vi "HFRR ADV v014 new software.vi"() -> ()   [LabVIEW 2025] (continued)
            }
          }
        }
        n1459 = VISA Flush I/O Buffer(VISA resource name=w1688) -> (VISA resource name out=w1679:refnum<visa-resource-name>, error out=→"error out 9":errorcluster)  [unwired: 2 in]
        "Port 2a" <- TRUE ("Port 2a")
      }
      frame Error {
        w1729 = u16 0 items=["None", "XON/XOFF", "RTS/CTS", "XON/XOFF & RTS/CTS", "DTR/DSR", "XON/XOFF & DTR/DSR"] ("flow control (0:none)  2")
        w1727 = u16 10 items=["1.0"=10, "1.5"=15, "2.0"=20] ("stop bits 2")
        w1725 = u16 0 items=["None", "Odd", "Even", "Mark", "Space"] ("parity 2")
        w1726 = u32 10000  # timeout (10sec)
        n1460 = VISA Clear(VISA resource name=w1721, error in (no error)=w1718) -> (VISA resource name out=w1720:refnum<visa-resource-name>, error out=w1719:errorcluster)
        n1461 = VISA Close(VISA resource name=w1720, error in (no error)=w1719) -> (error out=w1722:errorcluster)
        n1462 = call <vilib>:"Clear Errors.vi"("error in (no error)"=w1722) -> ()  [unwired: 5 in, 2 out]
        n1463 = local write "Port 2a"(FALSE ("Port 2a")) -> ()
        n1464 = local read "Com Port 2"() -> (w1715:refnum<visa-resource-name>)
        "visa due" <- w1715
        n1465 = call-poly "VISA Configure Serial Port"("VISA resource name"=w1715, "timeout (10sec)"=w1726, "baud rate (9600)"=u32 250000 ("baud rate  2"), "data bits (8)"=u16 8 ("data bits  2"), "parity (0:none)"=w1725, "stop bits (10: 1 bit)"=w1727, "flow control (0:none)"=w1729) -> ("VISA resource name out"=w1730:refnum<visa-resource-name>, "error out"=w1731:errorcluster)  [unwired: 7 in]
        n1466 = flat-sequence {
          tunnel: w1730 -> [w1733]
          tunnel: w1731 -> [w1732]
          tunnel: [w1733] -> w1723
          tunnel: [w1732] -> w1716
          frame #0 {
            n1467 = Wait (ms)(milliseconds to wait=u32 50) -> ()  [unwired: 1 out]
          }
        }
        "Residual Due" <- ""
        "Port 2 Error" <- w1716
      }
    }
    n1468 = local read "Quit"() -> (w1658:bool)
    "Error Due" <- w1663
  }
  n1469 = local write "FRICVALZ"(0.0 ("FRICVALZ")) -> ()
  n1470 = property on="RUN" class="Bool (strict)"("Visible"=TRUE) -> ()  [unwired: 2 in, 2 out]
  n1471 = while {
    tunnel: [w1750] -> _
    tunnel: [w1735] -> w54
    i -> [w1750]
    stop <- w1735 stop-if-true
    n1472 = local read "conststatus"() -> (w1739:dbl)
    n1473 = local read "Main Tab"() -> (w1737:T2)
    n1474 = local read "EDIT"() -> (w1756:bool)
    n1475 = local read "Rate"() -> (w1755:dbl)
    n1476 = case shown="True" w1756 {
      tunnel: [FALSE TRUE] -> w1742
      frame False {
      }
      frame True {
      }
    }
    n1477 = property on="Time slide" class="Slide (strict)"("Scale.Range:Maximum"=2500.0) -> ()  [unwired: 2 in, 2 out]
    n1478 = Equal?(x=w1737, y=T27."About" ("Main Tab")) -> (x = y?=w1748:bool)
    n1479 = Equal?(x=w1739, y=0.0) -> (x = y?=w1740:bool)
    n1480 = Divide(x=1.0, y=w1755) -> (x/y=w1751:dbl)
    "Time 2" <- w1751
    n1481 = case shown="True" w1740 {
      frame False {
      }
      frame True {
        # "C:\\WinDucom\\calibrate WO 2391.dcf"
        n1482 = local write "Lan flag"(22) -> ()
        n1483 = local write "conststatus"(10.0 ("rpm value : 2")) -> ()
        n1484 = String To Path(string="C:\\LAB-IQ\\calibrate WO 2465.dcf") -> (path=w1762:path)
        n1485 = Open/Create/Replace File "Open File"(file path (use dialog)=w1762) -> (refnum out=w1760:refnum<file>)  [unwired: 5 in, 2 out]
        n1486 = for {
          N: 23 -> [_]
          tunnel: w1760 -> [w1771]
          i -> [w1765]
          (unwired) TRUE ("line mode (F)")
          n1487 = Read from Text File "Read File"(file (use dialog)=w1771) -> (text=w1770:string)  [unwired: 3 in, 3 out]
          n1488 = Match Pattern(string=w1770, regular expression="]") -> (after substring=w1768:string)  [unwired: 1 in, 3 out]
          n1489 = String Subset(string=w1770, offset (0)=5, length (rest)=10 ("length (rest)")) -> (substring=w1763:string)
          n1490 = Fract/Exp String To Number(string=w1763) -> (number=w1764:dbl)  [unwired: 3 in, 1 out]
          n1491 = Match Pattern(string=w1768, regular expression="-") -> (before substring=w1766:string)  [unwired: 1 in, 3 out]
          n1492 = case shown="19" w1765 {
            tunnel: w1764 -> [w1774 w1775 w1776 w1777 _ _ _ w1782 w1783 _ w1784 w1785 w1786 w1787 w1788 w1789 _ w1790 w1791 _ _ _ _ _]
            tunnel: w1766 -> [_ _ _ _ w1778 w1779 w1780 _ _ _ _ _ _ _ _ _ _ _ _ w1792 w1793 w1794 w1795 _]
            frame 0 {
              n1493 = local write "FRIC. FORCE :"(w1774) -> ()
            }
            frame 1 {
              n1494 = local write "TEMPERATURE :"(w1775) -> ()
            }
            frame 2 {
              n1495 = local write "HUMIDITY:"(w1776) -> ()
            }
            frame 3 {
              n1496 = local write "AIR TEMPERATURE :"(w1777) -> ()
            }
            frame 4 {
              n1497 = local write "Com Port 1"(w1778) -> ()
            }
            frame 5 {
              n1498 = local write "Com Port 2"(w1779) -> ()
              n1499 = local write "visa due"(w1779) -> ()
            }
            frame 6 {
              n1500 = String To Path(string=w1780) -> (path=w1781:path)
              n1501 = local write "File Path"(w1781) -> ()
              "String" <- w1780
            }
            frame 7 {
              n1502 = local write "DISPLACEMENT :"(w1782) -> ()
            }
            frame 8 {
              n1503 = local write "STROKE GAIN :"(w1783) -> ()
            }
            frame 9 {
            }
            frame 10 {
              n1504 = local write "Language Selection"(w1784) -> ()
            }
            frame 11 {
              n1505 = local write "CH-POWER +"(w1785) -> ()
            }
            frame 12 {
              n1506 = local write "CH-POWER -"(w1786) -> ()
            }
            frame 13 {
              n1507 = local write "CH-HEATER"(w1787) -> ()
            }
            frame 14 {
              n1508 = local write "CH-HUMIDITY WET"(w1788) -> ()
            }
            frame 15 {
              n1509 = local write "CH-HUMIDITY DRY"(w1789) -> ()
            }
            frame 16 {
            }
            frame 17 {
              n1510 = local write "AIR TEMP INTERCEPT:"(w1790) -> ()
            }
            frame 18 {
              n1511 = local write "TEMP INTERCEPT:"(w1791) -> ()
            }
            frame 21 {
              n1512 = local write "S.NO"(w1792) -> ()
            }
            frame 22 {
              n1513 = local write "Com Port 3"(w1793) -> ()
            }
            frame 20 {
              n1514 = local write "Camera Port :"(w1794) -> ()
            }
            frame 19 {
              n1515 = local write "C3 :"(w1795) -> ()
            }
            frame 23, Default {
            }
          }
        }
      }
    }
    n1516 = Select(t=u32 2500 ("milliseconds to wait"), s=w1748, f=u32 500 ("milliseconds to wait")) -> (s? t:f=w1746:u32)
    n1517 = Multiply(x=w1751, y=w1746) -> (x*y=w1753:dbl)
    n1518 = property on="Time slide" class="Slide (strict)"("Visible"=w1742) -> ()  [unwired: 2 in, 2 out]
    n1519 = call "Elapsed Time2"("Time Target (s)"=w1753, "Auto Reset"=TRUE) -> ("Time has Elapsed"=w1743:bool)  [unwired: 10 in, 7 out]
    n1520 = case shown="True" w1743 {
      frame False {
      }
      frame True {
        n1521 = stacked-sequence {
          frame #0 {
            # "DATA PROCESSING"
            # "115 mV/N"
            n1522 = local read "Sample Temperature"() -> (w1798:dbl)
            n1523 = local read "RH Numeric:"() -> (w1805:dbl)
            n1524 = local read "HUMIDITY:"() -> (w1806:dbl)
            n1525 = local read "FRICVALZ"() -> (w1817:dbl)
            n1526 = local read "Friction"() -> (w1801:dbl)
            n1527 = Multiply(x=w1805, y=w1806) -> (x*y=→"Humidity ( %RH )" →"Hum" →"Hum 2":dbl)
            n1528 = call <vilib>:"Mean PtByPt.vi"("x"=w1798, "sample length"=100) -> ("mean"=w1797:dbl)  [unwired: 2 in, 1 out]
            "TEMP 2" <- w1797
            "TEMP 3" <- w1797
            n1529 = Subtract(x=w1801, y=w1817) -> (x-y=w1812:dbl)
            "FF 2" <- w1812
            "FF 4" <- w1812
            n1530 = local read "Ambient Temperature"() -> (→"AIR TEMP":dbl)
            n1531 = local read "TEMP"() -> (w1816:dbl)
            n1532 = local write "FF 3"(w1812) -> ()
            n1533 = Compound Arithmetic op=OR("FRICVALZ 4", "FRICVALZ 3", "FRICVALZ 2") -> (w1808:bool)
            n1534 = case shown="True" w1808 {
              tunnel: w1801 -> [_ w1823]
              frame False {
              }
              frame True {
                w1822 = FALSE ("FRICVALZ")
                n1535 = local write "FRICVALZ 3"(w1822) -> ()
                n1536 = local write "FRICVALZ 2"(w1822) -> ()
                n1537 = local write "FRICVALZ 4"(w1822) -> ()
                "FRICVALZ" <- w1823
              }
            }
            n1538 = Not A Number/Path/Refnum?(number/path/refnum=w1816) -> (NaN/Path/Refnum?=w1815:bool)
            n1539 = Not A Number/Path/Refnum?(number/path/refnum=w1812) -> (NaN/Path/Refnum?=w1814:bool)
            n1540 = Divide(x=w1812, y=1.96) -> (x/y=w1809:dbl)
            n1541 = Compound Arithmetic op=OR(w1815, w1814) -> (w1813:bool)
            n1542 = Not A Number/Path/Refnum?(number/path/refnum=w1809) -> (NaN/Path/Refnum?=w1810:bool)
            n1543 = case shown="True" w1813 {
              frame False {
              }
              frame True {
                n1544 = local write "TEMP"(0.0 ("TEMP")) -> ()
                n1545 = local write "FF 2"(0.0 ("FF 2")) -> ()
                n1546 = local write "reinit"(TRUE ("reinit")) -> ()
              }
            }
            n1547 = local write "TEMP"(w1797) -> ()
            n1548 = Select(t=0.0, s=w1810, f=w1809) -> (s? t:f=w1800:dbl)
            "COF 2" <- w1800
            n1549 = local write "COF 3"(w1800) -> ()
          }
        }
      }
    }
    n1550 = Wait (ms)(milliseconds to wait=u32 50) -> ()  [unwired: 1 out]
    n1551 = local read "Quit"() -> (w1735:bool)
    "Rate" <- 2500.0 ("No of Samples")
  }
  n1552 = while {
    tunnel: w57 -> [_]
    tunnel: [w1850] -> _
    tunnel: [w1826] -> w56
    i -> [w1850]
    stop <- w1826 stop-if-true
    # "C:\\LAB-IQ-NXT\\Scar View.exe"
    n1553 = local read "OK Button 16"() -> (w1839:bool)
    n1554 = local read "Main Tab"() -> (w1832:T2)
    n1555 = local read "service 3"() -> (w1833:bool)
    n1556 = local read "OPEN 6"() -> (w1835:bool)
    n1557 = local read "EDIT 2"() -> (w1837:bool)
    n1558 = flat-sequence {
      frame #0 {
        n1559 = local read "SAVE 2"() -> (w2452:bool)
        n1560 = stacked-sequence {
          frame #0 {
            n1561 = local read "EDIT"() -> (w2506:bool)
            n1562 = case shown="True" w2506 {
              tunnel: [u8 2 ("Disabled") u8 0 ("Disabled")] -> _
              frame False {
                w2508 = FALSE
                n1563 = local write "Password"("") -> ()
                n1564 = property on="SrvM CP" class="Bool (strict)"("Visible"=w2508) -> ()  [unwired: 2 in, 2 out]
                n1565 = property on="message" class="Str"("Visible"=w2508) -> ()  [unwired: 2 in, 2 out]
                n1566 = local write "x = y?"(w2508) -> ()
                n1567 = property on="Password" class="Str"("Visible"=w2508) -> ()  [unwired: 2 in, 2 out]
                n1568 = property on="ENTER THE NEW PASSWORD" class="Str"("Visible"=w2508) -> ()  [unwired: 2 in, 2 out]
                n1569 = property on="ENTER CURRENT PASSWORD" class="Str"("Visible"=w2508) -> ()  [unwired: 2 in, 2 out]
                n1570 = local write "SrvM CP"(w2508) -> ()
              }
              frame True {
                w2511 = TRUE
                n1571 = property on="SrvM CP" class="Bool (strict)"("Visible"=w2511) -> ()  [unwired: 2 in, 2 out]
                n1572 = property on="Password" class="Str"("Visible"=w2511) -> ()  [unwired: 2 in, 2 out]
              }
            }
            "dipl pwd" <- "@143$\n" ("dipl pwd")
          }
          frame #1 {
            # "Gain password"
            n1573 = String To Byte Array(string="ENTER CURRENT PASSWORD") -> (unsigned byte array=w2516:u8[])
            n1574 = Search 1D Array(1D array=w2516, element=u8 10) -> (index of element=w2519:i32)  [unwired: 1 in]
            n1575 = Index Array(array=w2516, index=w2519) -> (element=w2515:u8)
            n1576 = Equal?(x=w2515, y=10) -> (x = y?=w2513:bool)
            n1577 = case shown="True" w2513 {
              frame False {
                n1578 = property on="ENTER THE NEW PASSWORD" class="Str"("Visible"=FALSE) -> ()  [unwired: 2 in, 2 out]
              }
              frame True {
                # "password"
                # "change password logic"
                n1579 = local read "ENTER CURRENT PASSWORD"() -> (w2532:string)
                n1580 = local read "dipl pwd"() -> (w2526:string)
                n1581 = String To Byte Array(string=w2532) -> (unsigned byte array=w2534:u8[])
                n1582 = String To Byte Array(string=w2526) -> (unsigned byte array=w2527:u8[])
                n1583 = Array Size(array=w2534) -> (size(s)=w2531:i32)
                n1584 = Array Size(array=w2527) -> (size(s)=w2529:i32)
                n1585 = for {
                  N: w2531 -> [_]
                  tunnel: w2534 -> [w2558]
                  tunnel: [w2556] -> w2535 mode=indexing
                  tunnel: w2531 -> [w2550]
                  i -> [w2551]
                  n1586 = Decrement(x=w2550) -> (x-1=w2548:i32)
                  n1587 = Equal?(x=w2551, y=w2548) -> (x = y?=w2549:bool)
                  n1588 = Index Array(array=w2558, index=w2551) -> (element=w2552:u8)
                  n1589 = Number To Decimal String(number=w2552) -> (decimal integer string=w2557:string)  [unwired: 1 in]
                  n1590 = Select(t="", s=w2549, f="\r") -> (s? t:f=w2554:string)
                  n1591 = Concatenate Strings(w2557, w2554) -> (w2556:string)
                }
                n1592 = for {
                  N: w2529 -> [_]
                  tunnel: w2527 -> [w2546]
                  tunnel: [w2544] -> w2528 mode=indexing
                  tunnel: w2529 -> [w2541]
                  i -> [w2542]
                  n1593 = Decrement(x=w2541) -> (x-1=w2540:i32)
                  n1594 = Equal?(x=w2542, y=w2540) -> (x = y?=w2539:bool)
                  n1595 = Index Array(array=w2546, index=w2542) -> (element=w2545:u8)
                  n1596 = Number To Decimal String(number=w2545) -> (decimal integer string=w2543:string)  [unwired: 1 in]
                  n1597 = Select(t="", s=w2539, f="\r") -> (s? t:f=w2536:string)
                  n1598 = Concatenate Strings(w2543, w2536) -> (w2544:string)
                }
                n1599 = local read "string"() -> (w2533:string)
                n1600 = Concatenate Strings(w2528) -> (w2522:string)
                n1601 = Concatenate Strings(w2533) -> (w2530:string)
                n1602 = Concatenate Strings(w2535) -> (w2523:string)
                n1603 = Equal?(x=w2523, y=w2530) -> (x = y?=w2525:bool)
                n1604 = Equal?(x=w2523, y=w2522) -> (x = y?=w2521:bool)
                n1605 = Or(x=w2525, y=w2521) -> (x .or. y?=w2524:bool)
                n1606 = case shown="True" w2524 {
                  frame False {
                  }
                  frame True {
                    n1607 = property on="ENTER THE NEW PASSWORD" class="Str"("Visible"=TRUE) -> ()  [unwired: 2 in, 2 out]
                  }
                }
              }
            }
          }
          frame #2 {
            n1608 = String To Byte Array(string="ENTER THE NEW PASSWORD") -> (unsigned byte array=w2561:u8[])
            n1609 = Search 1D Array(1D array=w2561, element=u8 10) -> (index of element=w2565:i32)  [unwired: 1 in]
            n1610 = Index Array(array=w2561, index=w2565) -> (element=w2563:u8)
            n1611 = Equal?(x=w2563, y=10) -> (x = y?=w2560:bool)
            n1612 = case shown="False" w2560 {
              frame False {
              }
              frame True {
                n1613 = local write "EDIT"(FALSE) -> ()
                n1614 = local write "SrvM CP"(FALSE) -> ()
                n1615 = local read "ENTER THE NEW PASSWORD"() -> (w2568:string)
                n1616 = String To Byte Array(string=w2568) -> (unsigned byte array=w2573:u8[])
                n1617 = Array Size(array=w2573) -> (size(s)=w2570:i32)
                n1618 = for {
                  N: w2570 -> [_]
                  tunnel: w2573 -> [w2586]
                  tunnel: [w2583] -> w2575 mode=indexing
                  tunnel: w2570 -> [w2578]
                  i -> [w2576]
                  n1619 = Decrement(x=w2578) -> (x-1=w2579:i32)
                  n1620 = Equal?(x=w2576, y=w2579) -> (x = y?=w2580:bool)
                  n1621 = Index Array(array=w2586, index=w2576) -> (element=w2585:u8)
                  n1622 = Number To Decimal String(number=w2585) -> (decimal integer string=w2584:string)  [unwired: 1 in]
                  n1623 = Select(t="", s=w2580, f="\r") -> (s? t:f=w2577:string)
                  n1624 = Concatenate Strings(w2584, w2577) -> (w2583:string)
                }
                n1625 = local read "file path"() -> (w2567:path)
                n1626 = Concatenate Strings(w2575) -> (w2569:string)
                n1627 = Delete(path (use dialog)=w2567) -> (deleted path=w2571:path)  [unwired: 4 in, 2 out]
                n1628 = call <vilib>:"Write Characters To File.vi"("append to file? (new file:F)"=FALSE, "character string"=w2569, "file path (dialog if empty)"=w2571) -> ()  [unwired: 2 in, 1 out]
              }
            }
          }
          frame #3 {
            n1629 = case shown="True" "SrvM CP" {
              frame False {
                w2589 = ""
                n1630 = local write "ENTER CURRENT PASSWORD"(w2589) -> ()
                n1631 = local write "ENTER THE NEW PASSWORD"(w2589) -> ()
                n1632 = property on="ENTER CURRENT PASSWORD" class="Str"("Visible"=FALSE) -> ()  [unwired: 2 in, 2 out]
              }
              frame True {
                n1633 = property on="ENTER THE NEW PASSWORD" class="Str"() -> ("Visible"=w2590:bool)  [unwired: 2 in, 2 out]
                n1634 = Not(x=w2590) -> (.not. x?=w2591:bool)
                n1635 = property on="ENTER CURRENT PASSWORD" class="Str"("Visible"=w2591) -> ()  [unwired: 2 in, 2 out]
              }
            }
          }
          frame #4 {
            n1636 = String To Byte Array(string="Password") -> (unsigned byte array=w2598:u8[])
            n1637 = Search 1D Array(1D array=w2598, element=u8 10) -> (index of element=w2596:i32)  [unwired: 1 in]
            n1638 = Index Array(array=w2598, index=w2596) -> (element=w2597:u8)
            n1639 = Equal?(x=w2597, y=10) -> (x = y?=w2593:bool)
            n1640 = case shown="True" w2593 {
              frame False {
              }
              frame True {
                # "password"
                # "password"
                n1641 = local read "Password"() -> (w2611:string)
                n1642 = String To Byte Array(string=w2611) -> (unsigned byte array=w2614:u8[])
                n1643 = String To Byte Array(string="@143$\n") -> (unsigned byte array=w2600:u8[])
                n1644 = Array Size(array=w2614) -> (size(s)=w2609:i32)
                n1645 = Array Size(array=w2600) -> (size(s)=w2605:i32)
                n1646 = for {
                  N: w2609 -> [_]
                  tunnel: w2614 -> [w2648]
                  tunnel: [w2646] -> w2615 mode=indexing
                  tunnel: w2609 -> [w2643]
                  i -> [w2644]
                  n1647 = Decrement(x=w2643) -> (x-1=w2642:i32)
                  n1648 = Index Array(array=w2648, index=w2644) -> (element=w2647:u8)
                  n1649 = Equal?(x=w2644, y=w2642) -> (x = y?=w2641:bool)
                  n1650 = Number To Decimal String(number=w2647) -> (decimal integer string=w2645:string)  [unwired: 1 in]
                  n1651 = Select(t="", s=w2641, f="\r") -> (s? t:f=w2638:string)
                  n1652 = Concatenate Strings(w2645, w2638) -> (w2646:string)
                }
                n1653 = for {
                  N: w2605 -> [_]
                  tunnel: w2600 -> [w2659]
                  tunnel: [w2657] -> w2603 mode=indexing
                  tunnel: w2605 -> [w2654]
                  i -> [w2655]
                  n1654 = Decrement(x=w2654) -> (x-1=w2653:i32)
                  n1655 = Index Array(array=w2659, index=w2655) -> (element=w2658:u8)
                  n1656 = Equal?(x=w2655, y=w2653) -> (x = y?=w2652:bool)
                  n1657 = Number To Decimal String(number=w2658) -> (decimal integer string=w2656:string)  [unwired: 1 in]
                  n1658 = Select(t="", s=w2652, f="\r") -> (s? t:f=w2649:string)
                  n1659 = Concatenate Strings(w2656, w2649) -> (w2657:string)
                }
                n1660 = local read "file path"() -> (w2599:path)
                n1661 = call <vilib>:"Read Characters From File.vi"("file path (dialog if empty)"=w2599) -> ("character string"=w2613:string)  [unwired: 5 in, 3 out]
                "string" <- w2613
                n1662 = flat-sequence {
                  tunnel: [w2616] -> w2610
                  frame #0 {
                    w2616 = ""
                    n1663 = local write "Password"(w2616) -> ()
                  }
                }
                n1664 = Concatenate Strings(w2603) -> (w2604:string)
                n1665 = Concatenate Strings(w2613) -> (w2612:string)
                n1666 = Concatenate Strings(w2615) -> (w2607:string)
                n1667 = Equal?(x=w2607, y=w2612) -> (x = y?=w2602:bool)
                n1668 = Equal?(x=w2607, y=w2604) -> (x = y?=w2608:bool)
                n1669 = Or(x=w2602, y=w2608) -> (x .or. y?=w2601:bool)
                "x = y?" <- w2601
                n1670 = case shown="True" w2601 {
                  selector: w2601 -> [w2618 _]
                  tunnel: w2610 -> [_ _]
                  frame False {
                    n1671 = And(x=w2618, y=TRUE ("Visible")) -> (x .and. y?=w2619:bool)
                    n1672 = property on="message" class="Str"("Visible"=w2619) -> ()  [unwired: 2 in, 2 out]
                  }
                  frame True {
                    n1673 = control-ref of="This VI"() -> (w2630:refnum<vi>)
                    n1674 = property class="VI"(reference=w2630) -> (reference out=w2621:refnum<vi>, error out=w2625:errorcluster, "Panel"=w2629:refnum<vi>)  [unwired: 1 in]
                    n1675 = property on="message" class="Str"("Visible"=FALSE) -> ()  [unwired: 2 in, 2 out]
                    n1676 = property class="Pnl"(reference=w2629, error in=w2625) -> (reference out=w2623:refnum<vi>, error out=w2626:errorcluster, "Panes[]"=w2628:refnum<vi>[])
                    n1677 = for {
                      tunnel: w2628 -> [w2637] mode=indexing
                      tunnel: T21."Always On" ("Horizontal Scrollbar Visibility") -> [w2636]
                      tunnel: w2626 -> [w2633]
                      tunnel: [w2632] -> w2624
                      n1678 = property class="Pane"(reference=w2637, error in=w2633, "HorizScrollbarVisibility"=w2636) -> (reference out=w2634:refnum<vi>, error out=w2635:errorcluster)
                      n1679 = Close Reference(reference=w2634, error in (no error)=w2635) -> (error out=w2632:errorcluster)
                    }
                    n1680 = Close Reference(reference=w2623, error in (no error)=w2624) -> (error out=w2622:errorcluster)
                    n1681 = Close Reference(reference=w2621, error in (no error)=w2622) -> (error out=→"error out 6":errorcluster)
                  }
                }
              }
            }
          }
        }
        n1682 = local read "x = y?"() -> (w2458:bool)
        n1683 = local read "HUMIDITY: 2"() -> (w2460:dbl)
        n1684 = local read "HUMIDITY:"() -> (w2459:dbl)
        n1685 = property on="Port 2 Error" class="Clust (strict)"("Visible"="EDIT") -> ()  [unwired: 2 in, 2 out]
        n1686 = property on="Port 1 Error" class="Clust (strict)"("Visible"="EDIT") -> ()  [unwired: 2 in, 2 out]
        n1687 = case shown="True" "SrvM CP 2" {
          frame False {
          }
          frame True {
            n1688 = local write "SrvM CP 2"(FALSE ("SrvM CP 2")) -> ()
            n1689 = local read "HUMIDITY: 2"() -> (w2499:dbl)
            n1690 = local read "TEMP INTERCEPT: 2"() -> (w2498:dbl)
            n1691 = local read "DISPLACEMENT : 4"() -> (w2502:dbl)
            n1692 = local read "TEMPERATURE : 2"() -> (w2501:dbl)
            n1693 = local read "STROKE GAIN : 2"() -> (w2503:dbl)
            n1694 = local read "FRIC. FORCE : 2"() -> (w2504:dbl)
            n1695 = local read "AIR TEMP INTERCEPT: 2"() -> (w2497:dbl)
            n1696 = local read "AIR TEMPERATURE : 2"() -> (w2500:dbl)
            n1697 = local write "HUMIDITY:"(w2499) -> ()
            n1698 = local write "AIR TEMP INTERCEPT:"(w2498) -> ()
            n1699 = local write "TEMPERATURE :"(w2501) -> ()
            n1700 = local write "FRIC. FORCE :"(w2504) -> ()
            n1701 = local write "STROKE GAIN :"(w2503) -> ()
            n1702 = local write "DISPLACEMENT :"(w2502) -> ()
            n1703 = local write "AIR TEMPERATURE :"(w2500) -> ()
            n1704 = local write "TEMP INTERCEPT:"(w2497) -> ()
          }
        }
        n1705 = Or(x="SAVE", y=w2452) -> (x .or. y?=w2453:bool)
        n1706 = And(x="EDIT", y=w2458) -> (x .and. y?=w2456:bool)
        n1707 = local read "DISPLACEMENT : 4"() -> (w2469:dbl)
        n1708 = local read "TEMPERATURE : 2"() -> (w2467:dbl)
        n1709 = local read "STROKE GAIN : 2"() -> (w2473:dbl)
        n1710 = local read "DISPLACEMENT :"() -> (w2468:dbl)
        n1711 = local read "FRIC. FORCE : 2"() -> (w2476:dbl)
        n1712 = local read "TEMPERATURE :"() -> (w2465:dbl)
        n1713 = local read "STROKE GAIN :"() -> (w2472:dbl)
        n1714 = local read "FRIC. FORCE :"() -> (w2475:dbl)
        n1715 = case shown="True" w2456 {
          tunnel: [u8 2 ("Disabled") u8 0 ("Disabled")] -> w2455
          tunnel: [w2820 TRUE ("Visible")] -> w2454
          frame False {
            w2820 = FALSE ("Visible")
            n1716 = local write "EDIT 2"(w2820) -> ()
          }
          frame True {
          }
        }
        n1717 = case shown="True" w2453 {
          frame False {
          }
          frame True {
            n1718 = stacked-sequence {
              seq-local: [w2668 _ _] -> [_ w2815 _]
              frame #0 {
                (unwired) i16 5 ("precision (6)")
                # "[CH1]    - FF\n[CH2]   - TEMPERATURE\n[CH3]    - Humidity\n[CH4]    - AIR TEMP\n[CH5]\\- Visa Uno\n[CH6] \\- Visa Due\n[CH7]  \\- file path\n[CH8]   - Displacement Gain\n[CHA]   - Stroke Gain\n[CHB]   - Stroke PID Gain\n[CHC]   -Language Selection\n[CHD]   -Power +\n[CHE]   -Power_\n[CHF]   -Heater\n[CHG]   -Humidity Wet\n[CHH]   -Humidity Dry\n[CHI]   -Integral Time"
                n1719 = local read "Language Selection"() -> (w2716:enum16{"English", "Russian"})
                n1720 = local read "CH-HUMIDITY WET"() -> (w2674:u16)
                n1721 = local read "CH-HUMIDITY DRY"() -> (w2671:u16)
                n1722 = local read "STROKE GAIN :"() -> (w2660:dbl)
                n1723 = local read "CH-POWER +"() -> (w2683:u16)
                n1724 = local read "CH-POWER -"() -> (w2680:u16)
                n1725 = local read "CH-HEATER"() -> (w2677:u16)
                n1726 = local read "AIR TEMPERATURE :"() -> (w2663:dbl)
                n1727 = local read "DISPLACEMENT :"() -> (w2661:dbl)
                n1728 = local read "TEMPERATURE :"() -> (w2664:dbl)
                n1729 = local read "FRIC. FORCE :"() -> (w2665:dbl)
                n1730 = local read "HUMIDITY:"() -> (w2662:dbl)
                n1731 = Path To String(path="File Path") -> (string=w2732:string)
                n1732 = Number To Fractional String(number=w2660, width (-)=i16 10 ("precision (6)"), precision (6)=i16 5) -> (F-format string=w2723:string)  [unwired: 1 in]
                n1733 = Number To Fractional String(number=w2716, width (-)=i16 10 ("precision (6)"), precision (6)=i16 5) -> (F-format string=w2712:string)  [unwired: 1 in]
                n1734 = Number To Fractional String(number=w2683, width (-)=i16 10 ("precision (6)"), precision (6)=i16 5) -> (F-format string=w2706:string)  [unwired: 1 in]
                n1735 = Number To Fractional String(number=w2680, width (-)=i16 10 ("precision (6)"), precision (6)=i16 5) -> (F-format string=w2703:string)  [unwired: 1 in]
                n1736 = Number To Fractional String(number=w2677, width (-)=i16 10 ("precision (6)"), precision (6)=i16 5) -> (F-format string=w2698:string)  [unwired: 1 in]
                n1737 = Number To Fractional String(number=w2674, width (-)=i16 10 ("precision (6)"), precision (6)=i16 5) -> (F-format string=w2695:string)  [unwired: 1 in]
                n1738 = Number To Fractional String(number=w2671, width (-)=i16 10 ("precision (6)"), precision (6)=i16 5) -> (F-format string=w2690:string)  [unwired: 1 in]
                n1739 = local read "Com Port 1"() -> (w2667:refnum<visa-resource-name>)
                n1740 = local read "Com Port 2"() -> (w2666:refnum<visa-resource-name>)
                n1741 = Concatenate Strings(w2732, "\\" ("string")) -> (w2731:string)
                n1742 = Number To Fractional String(number=w2665, width (-)=i16 10 ("precision (6)"), precision (6)=i16 5) -> (F-format string=w2764:string)  [unwired: 1 in]
                n1743 = Number To Fractional String(number=w2664, width (-)=i16 10 ("precision (6)"), precision (6)=i16 5) -> (F-format string=w2763:string)  [unwired: 1 in]
                n1744 = Number To Fractional String(number=w2662, width (-)=i16 10 ("precision (6)"), precision (6)=i16 5) -> (F-format string=w2757:string)  [unwired: 1 in]
                n1745 = Number To Fractional String(number=w2663, width (-)=i16 10 ("precision (6)"), precision (6)=i16 5) -> (F-format string=w2751:string)  [unwired: 1 in]
                n1746 = Number To Fractional String(number=w2661, width (-)=i16 10 ("precision (6)"), precision (6)=i16 5) -> (F-format string=w2724:string)  [unwired: 1 in]
                n1747 = Concatenate Strings("[CHA]" ("string"), w2723, "- Stroke Gain" ("string"), "\r") -> (w2717:string)
                n1748 = Concatenate Strings("[CHC]" ("string"), w2712, "-Language Selection" ("string"), "\r") -> (w2709:string)
                n1749 = Concatenate Strings("[CHD]" ("string"), w2706, "-Power +" ("string"), "\r") -> (w2688:string)
                n1750 = Concatenate Strings("[CHG]" ("string"), w2695, "-Humidity Wet" ("string"), "\r") -> (w2685:string)
                n1751 = Concatenate Strings("[CHH]" ("string"), w2690, "-Humidity Dry" ("string"), "\r") -> (w2684:string)
                n1752 = Concatenate Strings("[CH1]" ("string"), w2764, " - FF" ("string"), "\r") -> (w2762:string)
                n1753 = Concatenate Strings("[CH2]" ("string"), w2763, " - TEMPERATURE" ("string"), "\r") -> (w2761:string)
                n1754 = Concatenate Strings("[CH3]" ("string"), w2757, " - Humidity" ("string"), "\r") -> (w2754:string)
                n1755 = Concatenate Strings("[CH4]" ("string"), w2751, " - AIR TEMP" ("string"), "\r") -> (w2747:string)
                n1756 = Concatenate Strings("[CH5]" ("string"), w2667, "- Visa Uno" ("string"), "\r") -> (w2740:string)
                n1757 = Concatenate Strings("[CH6]" ("string"), w2666, "- Visa Due" ("string"), "\r") -> (w2735:string)
                n1758 = Concatenate Strings("[CH7]" ("string"), w2731, "- file path" ("string"), "\r") -> (w2734:string)
                n1759 = Concatenate Strings("[CH8]" ("string"), w2724, "- Displacement Gain" ("string"), "\r") -> (w2727:string)
                n1760 = Concatenate Strings("[CHE]" ("string"), w2703, "-Power_" ("string"), "\r") -> (w2687:string)
                n1761 = Concatenate Strings("[CHF]" ("string"), w2698, "-Heater" ("string"), "\r") -> (w2686:string)
                n1762 = Concatenate Strings(w2762, w2761, w2754, w2747, w2740, w2735, w2734, w2727, w2717, w2709, w2688, w2687, w2686, w2685, w2684) -> (w2668:string)
                "gain" <- w2668
              }
              frame #1 {
                n1763 = local read "Camera Port :"() -> (w2776:string)
                n1764 = local read "C3 :"() -> (w2784:refnum<visa-resource-name>)
                n1765 = local read "TEMP INTERCEPT:"() -> (w2785:dbl)
                n1766 = local read "AIR TEMP INTERCEPT:"() -> (w2786:dbl)
                n1767 = local read "Com Port 3"() -> (w2787:refnum<visa-resource-name>)
                n1768 = Concatenate Strings("[CH8]" ("string"), w2776, "- Visa Camera" ("string"), "\r") -> (w2775:string)
                n1769 = Concatenate Strings("[CH7]" ("string"), w2784, "- Visa Humidity" ("string"), "\r") -> (w2780:string)
                n1770 = Number To Fractional String(number=w2785, width (-)=i16 10 ("precision (6)"), precision (6)=i16 5) -> (F-format string=w2803:string)  [unwired: 1 in]
                n1771 = Concatenate Strings("[CHL]" ("string"), w2787, "- Visa humid" ("string"), "\r") -> (w2790:string)
                n1772 = Number To Fractional String(number=w2786, width (-)=i16 10 ("precision (6)"), precision (6)=i16 5) -> (F-format string=w2810:string)  [unwired: 1 in]
                n1773 = Concatenate Strings("[CHK]" ("string"), w2803, "-TEMP INTERCEPT" ("string"), "\r") -> (w2799:string)
                n1774 = Concatenate Strings("[SNO]" ("string"), "S.NO", "-" ("string"), "\r") -> (w2795:string)
                n1775 = Concatenate Strings("[CHJ]" ("string"), w2810, "-AIR TEMP INTERCEPT" ("string"), "\r") -> (w2800:string)
                n1776 = String To Path(string="C:\\LAB-IQ\\calibrate WO 2465.dcf") -> (path=w2788:path)
                n1777 = Concatenate Strings(w2815, w2800, w2799, w2795, w2790, w2780, w2775) -> (w2814:string)
                n1778 = call <vilib>:"Write Characters To File.vi"("append to file? (new file:F)"=FALSE, "character string"=w2814, "file path (dialog if empty)"=w2788) -> ()  [unwired: 2 in, 1 out]
              }
              frame #2 {
                n1779 = local write "Lan flag"(0.0 ("Lan flag")) -> ()
                n1780 = local write "conststatus"(0.0 ("rpm value : 2")) -> ()
                n1781 = local write "SAVE"(FALSE ("OK Button 14")) -> ()
                n1782 = local write "SAVE 2"(FALSE ("SAVE 2")) -> ()
              }
            }
          }
        }
        n1783 = Subtract(x=w2460, y=w2459) -> (x-y=w2461:dbl)
        n1784 = local read "AIR TEMPERATURE : 2"() -> (w2464:dbl)
        n1785 = local read "AIR TEMPERATURE :"() -> (w2463:dbl)
        n1786 = Divide(x=w2461, y=w2459) -> (x/y=w2483:dbl)
        n1787 = Subtract(x=w2476, y=w2475) -> (x-y=w2474:dbl)
        n1788 = Subtract(x=w2467, y=w2465) -> (x-y=w2466:dbl)
        n1789 = Subtract(x=w2473, y=w2472) -> (x-y=w2471:dbl)
        n1790 = Subtract(x=w2469, y=w2468) -> (x-y=w2470:dbl)
        n1791 = Subtract(x=w2464, y=w2463) -> (x-y=w2462:dbl)
        n1792 = Divide(x=w2474, y=w2475) -> (x/y=w2494:dbl)
        n1793 = Divide(x=w2466, y=w2465) -> (x/y=w2487:dbl)
        n1794 = Divide(x=w2471, y=w2472) -> (x/y=w2491:dbl)
        n1795 = Divide(x=w2470, y=w2468) -> (x/y=w2490:dbl)
        n1796 = Multiply(x=w2483, y=100.0) -> (x*y=→"HUMIDITY  Calibration Error":dbl)
        n1797 = Divide(x=w2462, y=w2463) -> (x/y=w2486:dbl)
        n1798 = Multiply(x=w2494, y=100.0) -> (x*y=→"FRIC. FORCE Calibration Error":dbl)
        n1799 = Multiply(x=w2487, y=100.0) -> (x*y=→"TEMPERATURE  Calibration Error":dbl)
        n1800 = Multiply(x=w2491, y=100.0) -> (x*y=→"STROKE Calibration Error":dbl)
        n1801 = Multiply(x=w2490, y=100.0) -> (x*y=→"DISPLACEMENT  Calibration Error":dbl)
        n1802 = property on="EDIT 2" class="Bool (strict)"("Visible"=w2454) -> ()  [unwired: 2 in, 2 out]
        n1803 = property on="SAVE" class="Bool (strict)"("Visible"=w2454) -> ()  [unwired: 2 in, 2 out]
        n1804 = property on="SrvM CP" class="Bool (strict)"("Disabled"=w2455) -> ()  [unwired: 2 in, 2 out]
        n1805 = property on="visa due" class="CmbBox"("Disabled"=w2455) -> ()  [unwired: 2 in, 2 out]
        n1806 = property on="File Path" class="Path"("Disabled"=w2455) -> ()  [unwired: 2 in, 2 out]
        n1807 = Multiply(x=w2486, y=100.0) -> (x*y=→"AIR TEMPERATURE  Calibration Error":dbl)
        n1808 = property on="Language Selection" class="Enum (strict)"("Visible"=w2454) -> ()  [unwired: 2 in, 2 out]
        n1809 = property on="Tab Control 7" class="TabCtl (strict)"("Disabled"=w2455) -> ()  [unwired: 2 in, 2 out]
        n1810 = property on="AIR TEMP INTERCEPT:" class="DigNum (strict)"("Disabled"=w2455) -> ()  [unwired: 2 in, 2 out]
        n1811 = property on="CH-POWER -" class="DigNum (strict)"("Disabled"=w2455) -> ()  [unwired: 2 in, 2 out]
        n1812 = property on="CH-POWER +" class="DigNum (strict)"("Disabled"=w2455) -> ()  [unwired: 2 in, 2 out]
        n1813 = property on="AIR TEMPERATURE :" class="DigNum (strict)"("Disabled"=w2455) -> ()  [unwired: 2 in, 2 out]
        n1814 = property on="STROKE GAIN :" class="DigNum (strict)"("Disabled"=w2455) -> ()  [unwired: 2 in, 2 out]
        n1815 = property on="SPEED OUT:" class="DigNum (strict)"("Disabled"=w2455) -> ()  [unwired: 2 in, 2 out]
        n1816 = property on="CH-HUMIDITY DRY" class="DigNum (strict)"("Disabled"=w2455) -> ()  [unwired: 2 in, 2 out]
        n1817 = property on="HUMIDITY:" class="DigNum (strict)"("Disabled"=w2455) -> ()  [unwired: 2 in, 2 out]
        n1818 = property on="CH-HUMIDITY WET" class="DigNum (strict)"("Disabled"=w2455) -> ()  [unwired: 2 in, 2 out]
        n1819 = property on="TEMPERATURE :" class="DigNum (strict)"("Disabled"=w2455) -> ()  [unwired: 2 in, 2 out]
        n1820 = property on="DISPLACEMENT :" class="DigNum (strict)"("Disabled"=w2455) -> ()  [unwired: 2 in, 2 out]
        n1821 = property on="CH-HEATER" class="DigNum (strict)"("Disabled"=w2455) -> ()  [unwired: 2 in, 2 out]
        n1822 = property on="TEMP INTERCEPT:" class="DigNum (strict)"("Disabled"=w2455) -> ()  [unwired: 2 in, 2 out]
        n1823 = property on="FRIC. FORCE :" class="DigNum (strict)"("Disabled"=w2455) -> ()  [unwired: 2 in, 2 out]
      }
    }
    n1824 = local read "RUN"() -> (w1849:bool)
    n1825 = local read "RUN"() -> (w1847:bool)
    n1826 = disable-structure shown="Disabled" {
      disable-tunnel: [w1864 _] -> w1830
      disable-tunnel: [w1863 _] -> w1828
      frame Disabled {
        n1827 = local read "Temperature before test"() -> (w1857:dbl)
        n1828 = local read "Temperature after test"() -> (w1870:dbl)
        n1829 = case shown="True" "Save Results" {
          frame False {
          }
          frame True {
            w1886 = "\r"
            n1830 = local write "Save Results"(FALSE ("OK Button 5")) -> ()
            n1831 = local read "Temperature before test"() -> (w1924:dbl)
            n1832 = local read "Temperature after test"() -> (w1926:dbl)
            n1833 = local read "Humidity before test"() -> (w1923:dbl)
            n1834 = local read "Humidity after test"() -> (w1925:dbl)
            n1835 = local read "WS1.4"() -> (w1930:dbl)
            n1836 = local read "AVP"() -> (w1928:dbl)
            n1837 = Number To Fractional String(number=w1930, width (-)=i16 6, precision (6)=i16 1) -> (F-format string=w1890:string)  [unwired: 1 in]
            n1838 = local read "MWSD"() -> (w1927:dbl)
            n1839 = local read "String"() -> (w1919:string)
            n1840 = local read "FILE"() -> (w1922:string)
            n1841 = local read "HCF"() -> (w1929:dbl)
            n1842 = Number To Fractional String(number=w1923, width (-)=i16 6, precision (6)=i16 1) -> (F-format string=w1915:string)  [unwired: 1 in]
            n1843 = Number To Fractional String(number=w1924, width (-)=i16 6, precision (6)=i16 1) -> (F-format string=w1912:string)  [unwired: 1 in]
            n1844 = Number To Fractional String(number=w1925, width (-)=i16 6, precision (6)=i16 1) -> (F-format string=w1908:string)  [unwired: 1 in]
            n1845 = Number To Fractional String(number=w1926, width (-)=i16 6, precision (6)=i16 1) -> (F-format string=w1904:string)  [unwired: 1 in]
            n1846 = Number To Fractional String(number=w1928, width (-)=i16 6, precision (6)=i16 3) -> (F-format string=w1897:string)  [unwired: 1 in]
            n1847 = Concatenate Strings(w1919, w1922) -> (w1941:string)
            n1848 = Number To Fractional String(number=w1927, width (-)=i16 6, precision (6)=i16 1) -> (F-format string=w1901:string)  [unwired: 1 in]
            n1849 = Number To Fractional String(number=w1929, width (-)=i16 6, precision (6)=i16 2) -> (F-format string=w1895:string)  [unwired: 1 in]
            n1850 = Concatenate Strings("(" ("string"), w1890, ")Microns" ("string")) -> (w1889:string)
            n1851 = local read "REMARKS"() -> (w1921:string)
            "REMARKS 2" <- w1921
            n1852 = Concatenate Strings("(" ("string"), w1915, " ) % RH," ("string")) -> (w1916:string)
            n1853 = Concatenate Strings(w1895, ")" ("string")) -> (w1893:string)
            n1854 = Concatenate Strings("(" ("string"), w1912, ")  Deg C ," ("string")) -> (w1911:string)
            n1855 = Concatenate Strings("(" ("string"), w1908, " ) % RH," ("string")) -> (w1907:string)
            n1856 = Concatenate Strings("(" ("string"), w1904, ")  Deg C ," ("string")) -> (w1903:string)
            n1857 = Concatenate Strings("(" ("string"), w1901, ")  Microns," ("string")) -> (w1900:string)
            n1858 = Concatenate Strings("(" ("string"), w1897, ")  kPa," ("string")) -> (w1887:string)
            n1859 = Concatenate Strings(w1941, ".dwm" ("Substring")) -> (w1939:string)
            n1860 = String To Path(string=w1939) -> (path=w1938:path)
            n1861 = Concatenate Strings(w1921, w1886, " Humidity before test= " ("Substring"), w1916, w1886, " Temperature before test = " ("Substring"), w1911, w1886, " Humidity after test= " ("Substring"), w1907, w1886, "Temperature after test = " ("Substring"), w1903, w1886, "MSD = " ("Substring"), w1900, w1886, "  AVP = " ("Substring"), w1887, w1886, "  HCF                     =( " ("Substring"), w1893, w1886, " WS1.4                  = " ("Substring"), w1889, w1886) -> (w1885:string)
            "data" <- w1885
            n1862 = call <vilib>:"Write Characters To File.vi"("append to file? (new file:F)"=FALSE, "character string"=w1885, "file path (dialog if empty)"=w1938) -> ()  [unwired: 2 in, 1 out]
            n1863 = Match Pattern(string=w1885, regular expression="!") -> (after substring=→"export":string)  [unwired: 1 in, 3 out]
          }
        }
        n1864 = Add(x=231.864, y=w1857) -> (x+y=w1854:dbl)
        n1865 = Add(x=231.864, y=w1870) -> (x+y=w1867:dbl)
        n1866 = Divide(x=1705.984, y=w1854) -> (x/y=w1855:dbl)
        n1867 = Divide(x=1705.984, y=w1867) -> (x/y=w1868:dbl)
        n1868 = local read "Humidity before test"() -> (w1859:dbl)
        n1869 = local read "Humidity after test"() -> (w1872:dbl)
        n1870 = Subtract(x=8.017352 ("y"), y=w1855) -> (x-y=w1881:dbl)
        n1871 = Subtract(x=8.017352 ("y"), y=w1868) -> (x-y=w1875:dbl)
        n1872 = expression code="10**y"(w1881) -> (w1861:dbl)
        n1873 = expression code="10**y"(w1875) -> (w1874:dbl)
        n1874 = Multiply(x=w1859, y=w1861) -> (x*y=w1860:dbl)
        n1875 = Multiply(x=w1872, y=w1874) -> (x*y=w1873:dbl)
        n1876 = Divide(x=w1860, y=750.0) -> (x/y=w1876:dbl)
        n1877 = Divide(x=w1873, y=750.0) -> (x/y=w1877:dbl)
        n1878 = Add(x=w1876, y=w1877) -> (x+y=w1878:dbl)
        n1879 = Divide(x=w1878, y=2.0) -> (x/y=w1880:dbl)
        n1880 = local write "AVP"(w1880) -> ()
        n1881 = Subtract(x=1.4, y=w1880) -> (x-y=w1863:dbl)
        n1882 = local read "HCF"() -> (w1864:dbl)
      }
      frame Enabled {
      }
    }
    n1883 = case shown="True" "EDIT 3" {
      frame False {
      }
      frame True {
        n1884 = local write "EDIT 3"(FALSE ("EDIT 3")) -> ()
        n1885 = local write "Main Tab"(T2."About" ("Main Tab")) -> ()
      }
    }
    n1886 = case shown="False" w1849 {
      frame False {
        n1887 = local read "stopT"() -> (w2827:bool)
        n1888 = case shown="True" w2827 {
          frame False {
          }
          frame True {
            n1889 = local write "stopT"(FALSE) -> ()
          }
        }
      }
      frame True {
        "stopT" <- TRUE
      }
    }
    n1890 = case shown="False" w1847 {
      frame False {
      }
      frame True {
      }
    }
    n1891 = case shown="True" w1837 {
      frame False {
        n1892 = property on="Password 2" class="Str"("Visible"=FALSE) -> ()  [unwired: 2 in, 2 out]
        n1893 = local write "Password 2"("" ("Password")) -> ()
      }
      frame True {
        n1894 = property on="Password 2" class="Str"("Visible"=TRUE) -> ()  [unwired: 2 in, 2 out]
        n1895 = Equal?(x="Password 2", y="HFRR1234") -> (x = y?=w1969:bool)
        n1896 = case shown="True" w1969 {
          tunnel: "Password 2" -> [w1972 _]
          frame False {
            n1897 = String Length(string=w1972) -> (length=w1973:i32)
            n1898 = Greater Than 0?(x=w1973) -> (x > 0?=w1971:bool)
            n1899 = case shown="False" w1971 {
              frame False {
                n1900 = property on="Password 2" class="Str"("Caption.Text"="Password (Advance Setting)") -> ()  [unwired: 2 in, 2 out]
              }
              frame True {
                n1901 = property on="Password 2" class="Str"("Caption.Text"="Incorrect Password!") -> ()  [unwired: 2 in, 2 out]
              }
            }
          }
          frame True {
            n1902 = local write "EDIT 2"(FALSE ("EDIT 2")) -> ()
            n1903 = local write "Password 2"("" ("Password")) -> ()
            n1904 = local write "Main Tab"(T2."Advance" ("Main Tab")) -> ()
            n1905 = local write "Main Dashboard Buttons"(T1."Advance" ("Main Dashboard Buttons")) -> ()
          }
        }
      }
    }
    n1906 = case shown="True" "Prog Uno" {
      frame False {
      }
      frame True {
        n1907 = stacked-sequence {
          frame #0 {
            n1908 = Delete(path (use dialog)=path "C:/LAB-IQ-NXT/UNOCOMPILE.bat" ("working directory")) -> ()  [unwired: 4 in, 3 out]
          }
          frame #1 {
            n1909 = local read "Com Port 1"() -> (w2434:refnum<visa-resource-name>)
            n1910 = Concatenate Strings("cmd.exe /c \"mode " ("command line"), w2434, ":1200,n,8,1\"\n" ("command line")) -> (w2439:string)
            n1911 = Concatenate Strings(w2439, "CD\\\nCD WinDucom\navrdude -C avrdude.conf -v -patmega328p -carduino -P" ("command line"), w2434, " -b115200 -D -Uflash:w:UNO_V20.hex:i\n" ("command line"), "\r") -> (w2441:string)
            "STR" <- w2441
            n1912 = call <vilib>:"Write Characters To File.vi"("append to file? (new file:F)"=FALSE, "character string"=w2441, "file path (dialog if empty)"=path "C:/LAB-IQ/UNOCOMPILE.bat" ("working directory")) -> ()  [unwired: 2 in, 1 out]
          }
          frame #2 {
            n1913 = disable-structure shown="Disabled" {
              frame Disabled {
                w2445 = "cmd.exe  /c \"C:\\LAB-IQ-NXT\\UNOCOMPILE.bat\"" ("string")
                n1914 = local write "Prog Uno"(FALSE ("run minimized? (F)")) -> ()
                n1915 = call <vilib>:"System Exec.vi"("expected output size  (4096)"=u32 65535, "run minimized? (F)"=FALSE, "wait until completion? (T)"=TRUE ("run minimized? (F)"), "working directory"=path "C:/LAB-IQ-NXT", "standard input"=w2445, "command line"=w2445) -> ("error out"=w2444:errorcluster, "standard output"=→"String 42":string)  [unwired: 2 in, 2 out]
                "error out 3" <- w2444
                n1916 = flat-sequence {
                  tunnel: w2444 -> [_]
                  frame #0 {
                  }
                }
              }
              frame Enabled {
              }
            }
          }
        }
      }
    }
    n1917 = case shown="\"ISO 12156\"" "TEST STANDARD" {
      tunnel: [2.0 ("Set Temp") 0.0 ("Set Temp") 2.0 ("Set Temp") 0.0 ("Set Temp")] -> w1838
      frame "ASTM D6079", Default {
        w2391 = 50.0 ("Hz")
        w2392 = 53.0 ("Set Rh")
        w2394 = 1.0 ("Set Strk")
        w2393 = 60.0 ("Set Temp")
        # "astm hide"
        n1918 = local write "NORMAL LOAD"(200.0 ("NORMAL LOAD")) -> ()
        n1919 = local write "Set Strk"(w2394) -> ()
        n1920 = local write "Set Hz"(w2391) -> ()
        n1921 = local write "Set Temp"(w2393) -> ()
        n1922 = local write "Set Rh"(w2392) -> ()
        n1923 = local write "test time"(75.0 ("test time")) -> ()
        n1924 = local write "Set Stroke:"(w2394) -> ()
        n1925 = local write "Set Humidity:"(w2392) -> ()
        n1926 = local write "Set Frequency:"(w2391) -> ()
        n1927 = local write "Set Temperature:"(w2393) -> ()
        "Test Standard" <- "ASTM D6079" ("Test Standard 2")
      }
      frame "ISO 12156" {
        n1928 = local write "Set Strk"(1.0 ("Set Strk")) -> ()
        n1929 = local write "NORMAL LOAD"(200.0 ("NORMAL LOAD")) -> ()
        n1930 = local write "Set Temp"(60.0 ("Set Temp")) -> ()
        n1931 = local write "test time"(75.0 ("test time")) -> ()
        n1932 = local write "Set Hz"(50.0 ("Hz")) -> ()
        n1933 = local write "Set Rh"(53.0 ("Set Rh")) -> ()
      }
      frame "CEC F-096-A-06" {
        n1934 = local write "Set Strk"(1.0 ("Set Strk")) -> ()
        n1935 = local write "NORMAL LOAD"(200.0 ("NORMAL LOAD")) -> ()
        n1936 = local write "Set Temp"(60.0 ("Set Temp")) -> ()
        n1937 = local write "test time"(75.0 ("test time")) -> ()
        n1938 = local write "Set Hz"(50.0 ("Hz")) -> ()
        n1939 = local write "Set Rh"(53.0 ("Set Rh")) -> ()
      }
      frame "Custom" {
      }
    }
    n1940 = case shown="True" "Prog Due" {
      frame False {
      }
      frame True {
        n1941 = stacked-sequence {
          frame #0 {
            n1942 = Delete(path (use dialog)=path "C:/LAB-IQ/DUECOMPILE.bat" ("working directory")) -> ()  [unwired: 4 in, 3 out]
          }
          frame #1 {
            n1943 = disable-structure shown="Disabled" {
              frame Disabled {
                n1944 = local read "visa due"() -> (w2416:string)
                n1945 = Concatenate Strings("cmd.exe /c \"mode " ("command line"), w2416, ":1200,n,8,1\"\n" ("command line")) -> (w2421:string)
                n1946 = Concatenate Strings(w2421, "CD\\\nCD WinDucom\nTIMEOUT 1\n bossac.exe -i -d --port=" ("command line"), w2416, " -U false -e -w -v -b DUE.bin -R\n" ("command line"), "\r") -> (w2423:string)
                "concatenated string 2" <- w2423
                n1947 = call <vilib>:"Write Characters To File.vi"("append to file? (new file:F)"=FALSE, "character string"=w2423, "file path (dialog if empty)"=path "C:/LAB-IQ-NXT/DUECOMPILE.bat" ("working directory")) -> ()  [unwired: 2 in, 1 out]
              }
              frame Enabled {
              }
            }
          }
          frame #2 {
            # "C:\\LAB-IQ-NXT\\DUECOMPILE.bat"
            n1948 = disable-structure shown="Disabled" {
              frame Disabled {
                w2428 = "cmd.exe  /c \"C:\\LAB-IQ-NXT\\DUECOMPILE.bat\"" ("string")
                n1949 = call <vilib>:"System Exec.vi"("expected output size  (4096)"=u32 65535, "run minimized? (F)"=FALSE, "wait until completion? (T)"=TRUE ("run minimized? (F)"), "working directory"=path "C:/LAB-IQ-NXT", "standard input"=w2428, "command line"=w2428) -> ("error out"=w2427:errorcluster, "standard output"=→"String 44":string)  [unwired: 2 in, 2 out]
                "error out 4" <- w2427
                n1950 = flat-sequence {
                  tunnel: w2427 -> [_]
                  frame #0 {
                  }
                }
              }
              frame Enabled {
              }
            }
            n1951 = local write "Prog Due"(FALSE ("Prog Due")) -> ()
          }
        }
      }
    }
    n1952 = Or(x=w1835, y=w1833) -> (x .or. y?=w1834:bool)
    n1953 = case shown="\"About\"" w1832 {
      tunnel: [T27."Acquire" ("Main Tab") T27."Compare Files" ("Main Tab") T27."About" ("Main Tab")] -> w1845
      frame "Acquire", Default {
      }
      frame "Compare Files" {
      }
      frame "About" {
      }
    }
    n1954 = Or(x=w1839, y="OPEN") -> (x .or. y?=w1840:bool)
    n1955 = case shown="True" w1840 {
      tunnel: w1839 -> [_ w1980]
      frame False {
      }
      frame True {
        n1956 = stacked-sequence {
          tunnel: w1980 -> [_ w2047 _ _]
          frame #0 {
            w1996 = "  " ("String 6")
            n1957 = local write "OPEN"(FALSE ("open")) -> ()
            n1958 = local read "string1 2"() -> (w1984:string)
            n1959 = local read "string1 3"() -> (w1983:string)
            n1960 = local read "string1 4"() -> (w1982:string)
            n1961 = property on="OPEN" class="Bool (strict)"("Visible"=FALSE) -> ()  [unwired: 2 in, 2 out]
            n1962 = local write "String 6"(w1996) -> ()
            n1963 = local write "String 7"(w1996) -> ()
            n1964 = local write "String 8"(w1996) -> ()
            n1965 = local write "String 12"(w1996) -> ()
            n1966 = local read "OK Button 16"() -> (w1981:bool)
            n1967 = String To Path(string=w1984) -> (path=w1992:path)
            n1968 = String To Path(string=w1983) -> (path=w1991:path)
            n1969 = String To Path(string=w1982) -> (path=w1990:path)
            n1970 = case shown="True" w1981 {
              tunnel: [w1997 w1998] -> w1985
              frame False {
                n1971 = local read "string1"() -> (w1997:string)
              }
              frame True {
                n1972 = local read "String Indicator 4"() -> (w1998:string)
              }
            }
            n1973 = Open/Create/Replace File "Open File"(file path (use dialog)=w1992) -> (refnum out=w1988:refnum<file>)  [unwired: 5 in, 2 out]
            n1974 = Open/Create/Replace File "Open File"(file path (use dialog)=w1991) -> (refnum out=w1987:refnum<file>)  [unwired: 5 in, 2 out]
            n1975 = Open/Create/Replace File "Open File"(file path (use dialog)=w1990) -> (refnum out=w1986:refnum<file>)  [unwired: 5 in, 2 out]
            n1976 = while {
              tunnel: w1988 -> [w2010]
              i -> [w2006]
              stop <- w2005 continue-if-true
              (unwired) TRUE ("line mode (F)")
              n1977 = Read from Text File "Read File"(file (use dialog)=w2010) -> (text=w2007:string)  [unwired: 3 in, 3 out]
              n1978 = local write "Numeric 11"(w2006) -> ()
              n1979 = String Length(string=w2007) -> (length=w2009:i32)
              n1980 = Greater?(x=w2009, y=1) -> (0:w2005:bool)
            }
            n1981 = while {
              tunnel: w1987 -> [w2016]
              i -> [w2012]
              stop <- w2011 continue-if-true
              (unwired) TRUE ("line mode (F)")
              n1982 = Read from Text File "Read File"(file (use dialog)=w2016) -> (text=w2013:string)  [unwired: 3 in, 3 out]
              n1983 = local write "Numeric 12"(w2012) -> ()
              n1984 = String Length(string=w2013) -> (length=w2015:i32)
              n1985 = Greater?(x=w2015, y=1) -> (0:w2011:bool)
            }
            n1986 = while {
              tunnel: w1986 -> [w2022]
              i -> [w2018]
              stop <- w2017 continue-if-true
              (unwired) TRUE ("line mode (F)")
              n1987 = Read from Text File "Read File"(file (use dialog)=w2022) -> (text=w2019:string)  [unwired: 3 in, 3 out]
              n1988 = local write "Numeric 13"(w2018) -> ()
              n1989 = String Length(string=w2019) -> (length=w2021:i32)
              n1990 = Greater?(x=w2021, y=1) -> (0:w2017:bool)
            }
            n1991 = String To Path(string=w1985) -> (path=w1993:path)
            n1992 = Open/Create/Replace File "Open File"(file path (use dialog)=w1993) -> (refnum out=w1989:refnum<file>)  [unwired: 5 in, 2 out]
            n1993 = while {
              tunnel: w1989 -> [w2004]
              i -> [w2000]
              stop <- w1999 continue-if-true
              (unwired) TRUE ("line mode (F)")
              n1994 = Read from Text File "Read File"(file (use dialog)=w2004) -> (text=w2001:string)  [unwired: 3 in, 3 out]
              n1995 = local write "Numeric 8"(w2000) -> ()
              n1996 = String Length(string=w2001) -> (length=w2003:i32)
              n1997 = Greater?(x=w2003, y=1) -> (0:w1999:bool)
            }
          }
          frame #1 {
            w2174 = FALSE ("ACTUAL   MERGE")
            # "Sample Temp"
            # "ECR"
            # "COF"
            # "Time\nCOF\nFF\nTemp"
            n1998 = case shown="True" w2047 {
              tunnel: [w2194 w2195] -> w2048
              frame False {
                n1999 = local read "string1"() -> (w2194:string)
              }
              frame True {
                n2000 = local read "String Indicator 4"() -> (w2195:string)
              }
            }
            n2001 = local read "string1 3"() -> (w2092:string)
            n2002 = String To Path(string=w2048) -> (path=w2179:path)
            n2003 = String To Path(string=w2092) -> (path=w2190:path)
            n2004 = local read "Numeric 12"() -> (w2176:i32)
            n2005 = local read "Numeric 8"() -> (w2178:i32)
            n2006 = local read "string1 2"() -> (w2093:string)
            n2007 = local read "string1 4"() -> (w2091:string)
            n2008 = Open/Create/Replace File "Open File"(file path (use dialog)=w2179) -> (refnum out=w2193:refnum<file>, error out=w2192:errorcluster)  [unwired: 5 in, 1 out]
            n2009 = Open/Create/Replace File "Open File"(file path (use dialog)=w2190) -> (refnum out=w2186:refnum<file>, error out=w2187:errorcluster)  [unwired: 5 in, 1 out]
            n2010 = for {
              N: w2178 -> [_]
              tunnel: w2193 -> [w2341]
              tunnel: w2192 -> [w2340]
              tunnel: [w2330] -> w2105 mode=indexing
              tunnel: [w2328] -> w2162 mode=indexing
              tunnel: [w2329] -> w2157 mode=indexing
              tunnel: w2174 -> [_]
              tunnel: [w2322] -> w2159 mode=indexing
              tunnel: [w2318] -> w2128 mode=indexing
              tunnel: [w2314] -> w2103 mode=indexing
              tunnel: [w2310] -> w2084 mode=indexing
              tunnel: [w2305] -> w2044 mode=indexing
              (unwired) TRUE ("line mode (F)")
              # "freq"
              # "Stroke"
              # "Time"
              # "CoF"
              # "Humidity"
              # "Temp"
              # "Air Temp"
              # "ECR"
              n2011 = Read from Text File "Read File"(file (use dialog)=w2341, error in=w2340) -> (text=w2306:string)  [unwired: 2 in, 3 out]
              n2012 = local write "String 6"(w2306) -> ()
              n2013 = String Subset(string=w2306, offset (0)=0, length (rest)=14 ("length (rest)")) -> (substring=w2334:string)
              n2014 = String Subset(string=w2306, offset (0)=35, length (rest)=9 ("length (rest)")) -> (substring=w2331:string)
              n2015 = String Subset(string=w2306, offset (0)=15, length (rest)=9 ("length (rest)")) -> (substring=w2337:string)
              n2016 = Fract/Exp String To Number(string=w2334) -> (number=w2330:dbl)  [unwired: 3 in, 1 out]
              n2017 = Fract/Exp String To Number(string=w2331) -> (number=w2329:dbl)  [unwired: 3 in, 1 out]
              n2018 = Fract/Exp String To Number(string=w2337) -> (number=w2328:dbl)  [unwired: 3 in, 1 out]
              n2019 = String Subset(string=w2306, offset (0)=85, length (rest)=9 ("length (rest)")) -> (substring=w2307:string)
              n2020 = String Subset(string=w2306, offset (0)=25, length (rest)=9 ("length (rest)")) -> (substring=w2313:string)
              n2021 = String Subset(string=w2306, offset (0)=55, length (rest)=9 ("length (rest)")) -> (substring=w2315:string)
              n2022 = String Subset(string=w2306, offset (0)=45, length (rest)=9 ("length (rest)")) -> (substring=w2321:string)
              n2023 = String Subset(string=w2306, offset (0)=65, length (rest)=9 ("length (rest)")) -> (substring=w2327:string)
              n2024 = Fract/Exp String To Number(string=w2313) -> (number=w2310:dbl)  [unwired: 3 in, 1 out]
              n2025 = Fract/Exp String To Number(string=w2307) -> (number=w2305:dbl)  [unwired: 3 in, 1 out]
              n2026 = Fract/Exp String To Number(string=w2315) -> (number=w2314:dbl)  [unwired: 3 in, 1 out]
              n2027 = Fract/Exp String To Number(string=w2321) -> (number=w2318:dbl)  [unwired: 3 in, 1 out]
              n2028 = Fract/Exp String To Number(string=w2327) -> (number=w2324:dbl)  [unwired: 3 in, 1 out]
              n2029 = Add(x=w2324, y=0.0) -> (x+y=w2322:dbl)
            }
            n2030 = for {
              N: w2176 -> [_]
              tunnel: w2187 -> [w2267]
              tunnel: w2186 -> [w2266]
              tunnel: [w2256] -> w2145 mode=indexing
              tunnel: [w2254] -> w2143 mode=indexing
              tunnel: [w2255] -> w2139 mode=indexing
              tunnel: w2174 -> [_]
              tunnel: [w2248] -> w2141 mode=indexing
              tunnel: [w2244] -> w2123 mode=indexing
              tunnel: [w2240] -> w2099 mode=indexing
              tunnel: [w2237] -> w2080 mode=indexing
              tunnel: [w2233] -> w2039 mode=indexing
              (unwired) 9 ("length (rest)")
              (unwired) 9 ("length (rest)")
              (unwired) TRUE ("line mode (F)")
              n2031 = Read from Text File "Read File"(file (use dialog)=w2266, error in=w2267) -> (text=w2234:string)  [unwired: 2 in, 3 out]
              n2032 = local write "String 8"(w2234) -> ()
              n2033 = String Subset(string=w2234, offset (0)=85) -> (substring=w2236:string)  [unwired: 1 in]
              n2034 = String Subset(string=w2234, offset (0)=35, length (rest)=9 ("length (rest)")) -> (substring=w2257:string)
              n2035 = String Subset(string=w2234, offset (0)=55, length (rest)=9 ("length (rest)")) -> (substring=w2242:string)
              n2036 = String Subset(string=w2234, offset (0)=25) -> (substring=w2238:string)  [unwired: 1 in]
              n2037 = String Subset(string=w2234, offset (0)=15, length (rest)=9 ("length (rest)")) -> (substring=w2263:string)
              n2038 = String Subset(string=w2234, offset (0)=0, length (rest)=14 ("length (rest)")) -> (substring=w2260:string)
